vi "No_____Auto_Routine_LeftTrialPieceTRAJ.vi"   [LabVIEW 2023]
uses:
  Shoulder/ShoulderGetSetpointEnum.ctl
  Trajectory/TrajectoryGlobals.vi
  <vilib>/Rock Robotics/WPI/ThirdParty/JAS_Junk/TrajLib/Trajectory_Library.lvlib
types:
  T1 = typedef "ShoulderGetSetpointEnum.ctl" = enum16{"ShoulderRest", "ShoulderShoot", "ShoulderAmp", "ArmFloorPickup", "ArmAmpDeposit", "ArmSpeakerShoot", "ArmStartPosition", "ArmRestPosition", "ArmSourceIntake", "ArmAwayShoot"}
  T2 = typedef "Trajectory_Library.lvlib/TRAJECTORY.ctl" = cluster{"TotalTImeSecs":dbl, "States":T3[]}
  T3 = typedef "Trajectory_Library.lvlib/TRAJ_STATE.ctl" = cluster{"TimeSeconds":dbl, "Velocity":dbl, "Acceleration":dbl, "POSE":T4, "Curvature":dbl}
  T4 = typedef "Trajectory_Library.lvlib/POSE2D.ctl" = cluster{"TRANSLATION":T5, "ROTATION":T6}
  T5 = typedef "Trajectory_Library.lvlib/TRANSLATION2D.ctl" = cluster{"X":dbl, "Y":dbl}
  T6 = typedef "Trajectory_Library.lvlib/ROTATION2D.ctl" = cluster{"VALUE":dbl, "COS":dbl, "SIN":dbl}
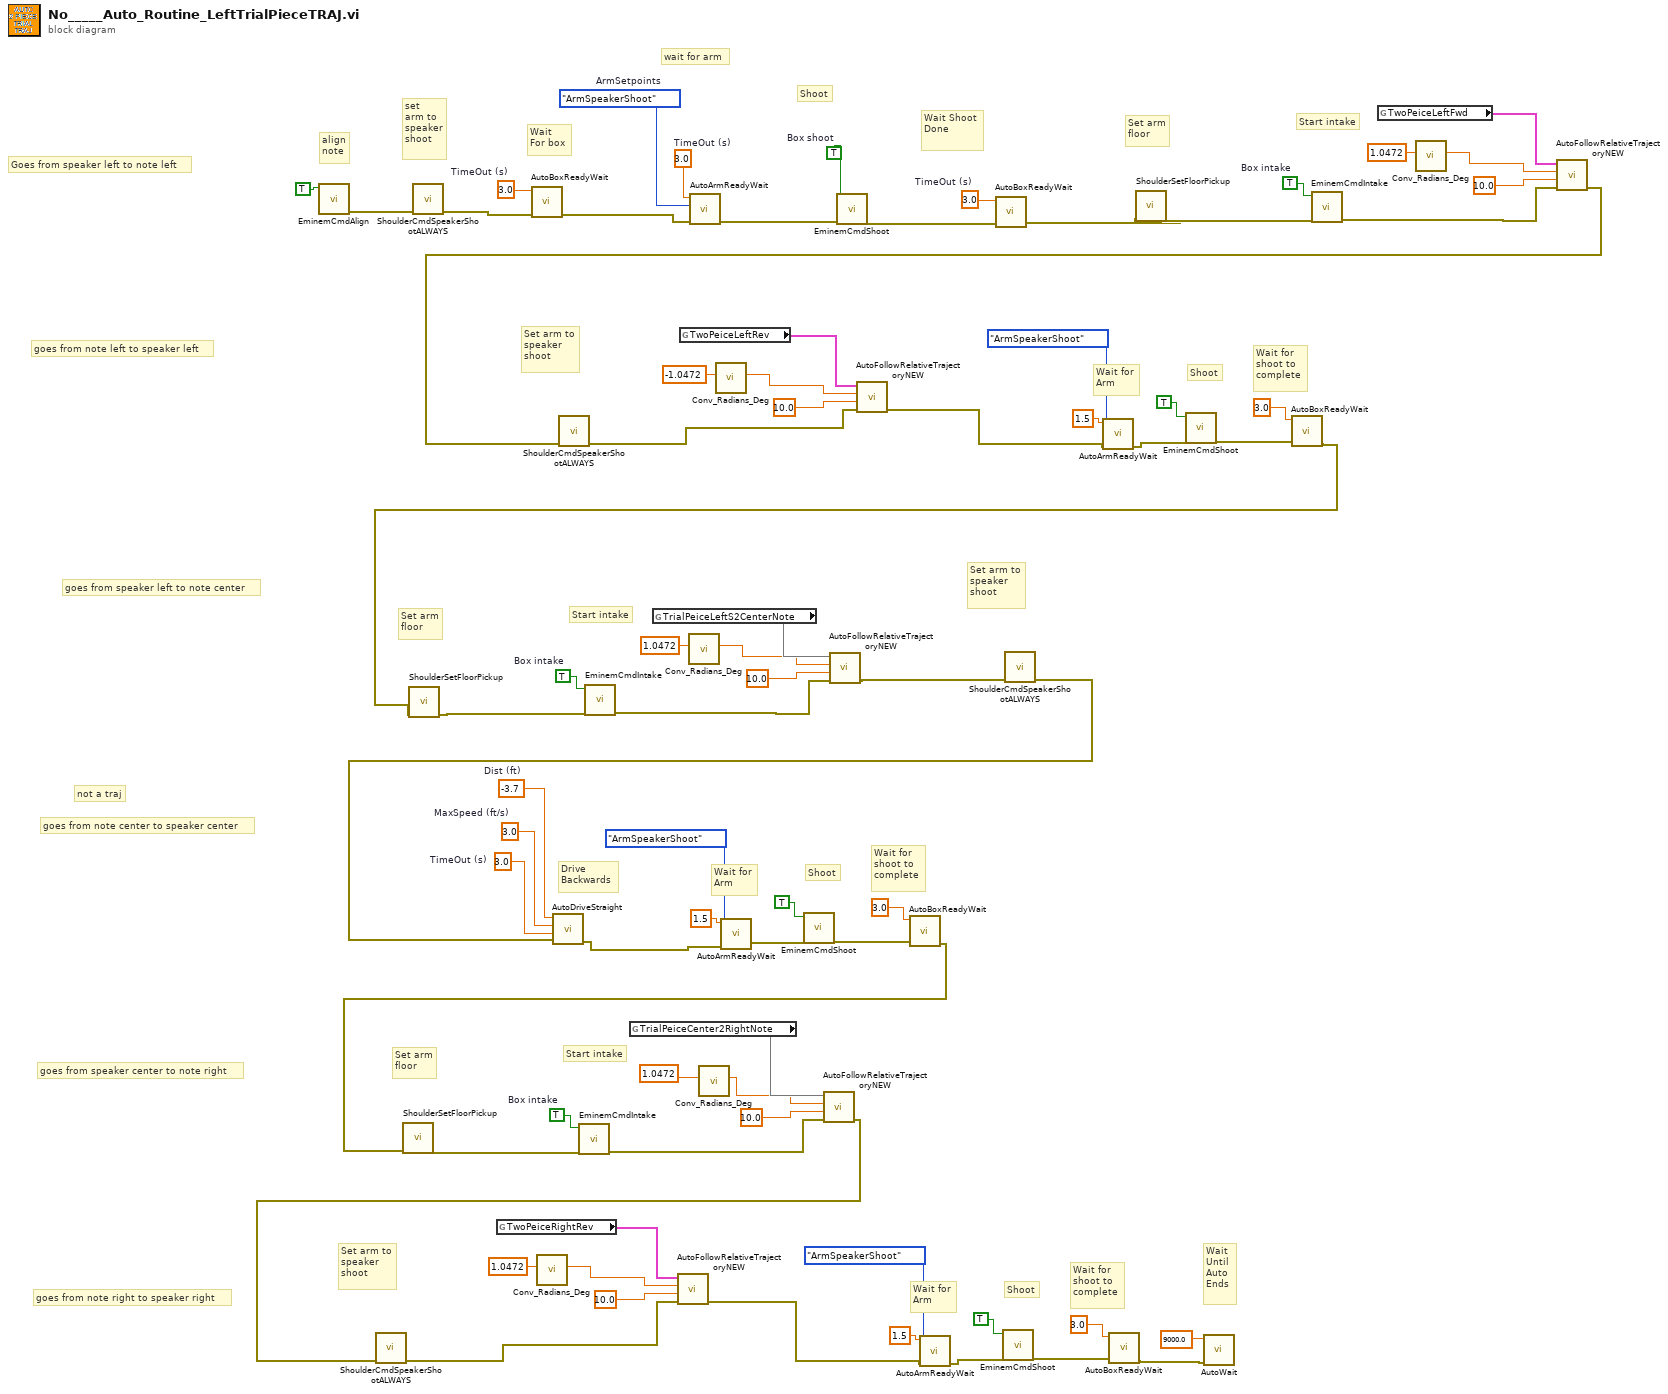
[diagram p0: block diagram]
diagram:
  w23 = TRUE  # Box intake
  w31 = 3.0  # TimeOut (s)
  w30 = 3.0  # MaxSpeed (ft/s)
  w29 = -3.7  # Dist (ft)
  w43 = TRUE  # Box intake
  w65 = 3.0  # TimeOut (s)
  w75 = TRUE  # Box intake
  w74 = TRUE  # Box shoot
  w73 = ShoulderGetSetpointEnum."ArmSpeakerShoot"  # ArmSetpoints
  w72 = 3.0  # TimeOut (s)
  w68 = 3.0  # TimeOut (s)
  # "Wait\nUntil\nAuto \nEnds"
  # "Wait for\nshoot to\ncomplete"
  # "Shoot"
  # "Wait for\nArm"
  # "Set arm to\nspeaker \nshoot"
  # "Start intake"
  # "Set arm\nfloor"
  # "not a traj"
  # "Wait for\nshoot to\ncomplete"
  # "Shoot"
  # "Wait for\nArm"
  # "Drive\nBackwards"
  # "Set arm to\nspeaker \nshoot"
  # "Start intake"
  # "Set arm\nfloor"
  # "goes from note right to speaker right"
  # "goes from speaker center to note right"
  # "goes from note center to speaker center"
  # "goes from speaker left to note center"
  # "goes from note left to speaker left"
  # "Goes from speaker left to note left"
  # "Wait for\nshoot to\ncomplete"
  # "Shoot"
  # "Wait for\nArm"
  # "Set arm to\nspeaker \nshoot"
  # "Start intake"
  # "Set arm\nfloor"
  # "Wait Shoot\nDone"
  # "Shoot"
  # "Wait\nFor box"
  # "set \narm to\nspeaker\nshoot"
  # "align\nnote"
  # "wait for arm"
  n1 = call "EminemCmdAlign.vi"("box align"=TRUE) -> ("error out"=w66:errorcluster)  [unwired: 10 in]
  n2 = call "ShoulderCmdSpeakerShootALWAYS.vi"("error in (no error)"=w66) -> ("error out"=w64:errorcluster)  [unwired: 10 in]
  n3 = global read "TrajectoryGlobals.vi" "TwoPeiceRightRev"() -> (w8:T2)
  n4 = call "AutoBoxReadyWait.vi"("error in (no error)"=w64, "TimeOut (s)"=w65) -> ("error out"=w63:errorcluster)  [unwired: 9 in]
  n5 = call <vilib>:"Conv_Radians_Deg.vi"("Radians"=1.0472) -> ("Degrees"=w6:dbl)  [unwired: 10 in]
  n6 = global read "TrajectoryGlobals.vi" "TrialPeiceCenter2RightNote"() -> (w20)
  n7 = global read "TrajectoryGlobals.vi" "TrialPeiceLeftS2CenterNote"() -> (w41)
  n8 = global read "TrajectoryGlobals.vi" "TwoPeiceLeftRev"() -> (w49:T2)
  n9 = call <vilib>:"Conv_Radians_Deg.vi"("Radians"=1.0472) -> ("Degrees"=w39:dbl)  [unwired: 10 in]
  n10 = call "AutoArmReadyWait.vi"("error in (no error)"=w63, "ArmSetpoints"=w73, "TimeOut (s)"=w72) -> ("error out"=w69:errorcluster)  [unwired: 8 in]
  n11 = call <vilib>:"Conv_Radians_Deg.vi"("Radians"=1.0472) -> ("Degrees"=w18:dbl)  [unwired: 10 in]
  n12 = call <vilib>:"Conv_Radians_Deg.vi"("Radians"=-1.0472) -> ("Degrees"=w47:dbl)  [unwired: 10 in]
  n13 = call "EminemCmdShoot.vi"("error in (no error)"=w69, 11:w74) -> ("error out"=w70:errorcluster)  [unwired: 9 in]
  n14 = call "AutoBoxReadyWait.vi"("error in (no error)"=w70, "TimeOut (s)"=w68) -> ("error out"=w62:errorcluster)  [unwired: 9 in]
  n15 = call "ShoulderSetFloorPickup.vi"("error in (no error)"=w62) -> ("error out"=w71:errorcluster)  [unwired: 10 in]
  n16 = call "EminemCmdIntake.vi"("error in (no error)"=w71, "Box intake"=w75) -> ("error out"=w61:errorcluster)  [unwired: 9 in]
  n17 = global read "TrajectoryGlobals.vi" "TwoPeiceLeftFwd"() -> (w60:T2)
  n18 = call <vilib>:"Conv_Radians_Deg.vi"("Radians"=1.0472) -> ("Degrees"=w58:dbl)  [unwired: 10 in]
  n19 = call "AutoFollowRelativeTrajectoryNEW.vi"("error in (no error)"=w61, "TimeOut (s)"=10.0, "End Orientation"=w58, "Trajectory"=w60) -> ("error out"=w56:errorcluster)  [unwired: 7 in]
  n20 = call "ShoulderCmdSpeakerShootALWAYS.vi"("error in (no error)"=w56) -> ("error out"=w45:errorcluster)  [unwired: 10 in]
  n21 = call "AutoFollowRelativeTrajectoryNEW.vi"("error in (no error)"=w45, "TimeOut (s)"=10.0, "End Orientation"=w47, "Trajectory"=w49) -> ("error out"=w44:errorcluster)  [unwired: 7 in]
  n22 = call "AutoArmReadyWait.vi"("error in (no error)"=w44, "ArmSetpoints"=ShoulderGetSetpointEnum."ArmSpeakerShoot", "TimeOut (s)"=1.5) -> ("error out"=w51:errorcluster)  [unwired: 8 in]
  n23 = call "EminemCmdShoot.vi"("error in (no error)"=w51, 11:TRUE ("Box shoot")) -> ("error out"=w54:errorcluster)  [unwired: 9 in]
  n24 = call "AutoBoxReadyWait.vi"("error in (no error)"=w54, "TimeOut (s)"=3.0) -> ("error out"=w36:errorcluster)  [unwired: 9 in]
  n25 = call "ShoulderSetFloorPickup.vi"("error in (no error)"=w36) -> ("error out"=w37:errorcluster)  [unwired: 10 in]
  n26 = call "EminemCmdIntake.vi"("error in (no error)"=w37, "Box intake"=w43) -> ("error out"=w42:errorcluster)  [unwired: 9 in]
  n27 = call "AutoFollowRelativeTrajectoryNEW.vi"("error in (no error)"=w42, "TimeOut (s)"=10.0, "End Orientation"=w39, "Trajectory"=w41) -> ("error out"=w35:errorcluster)  [unwired: 7 in]
  n28 = call "ShoulderCmdSpeakerShootALWAYS.vi"("error in (no error)"=w35) -> ("error out"=w24:errorcluster)  [unwired: 10 in]
  n29 = call "AutoDriveStraight.vi"("error in (no error)"=w24, "TimeOut (s)"=w31, "MaxSpeed (ft/s)"=w30, "Dist (ft)"=w29) -> ("error out"=w32:errorcluster)  [unwired: 7 in]
  n30 = call "AutoArmReadyWait.vi"("error in (no error)"=w32, "ArmSetpoints"=ShoulderGetSetpointEnum."ArmSpeakerShoot", "TimeOut (s)"=1.5) -> ("error out"=w26:errorcluster)  [unwired: 8 in]
  n31 = call "EminemCmdShoot.vi"("error in (no error)"=w26, 11:TRUE ("Box shoot")) -> ("error out"=w33:errorcluster)  [unwired: 9 in]
  n32 = call "AutoBoxReadyWait.vi"("error in (no error)"=w33, "TimeOut (s)"=3.0) -> ("error out"=w16:errorcluster)  [unwired: 9 in]
  n33 = call "ShoulderSetFloorPickup.vi"("error in (no error)"=w16) -> ("error out"=w22:errorcluster)  [unwired: 10 in]
  n34 = call "EminemCmdIntake.vi"("error in (no error)"=w22, "Box intake"=w23) -> ("error out"=w21:errorcluster)  [unwired: 9 in]
  n35 = call "AutoFollowRelativeTrajectoryNEW.vi"("error in (no error)"=w21, "TimeOut (s)"=10.0, "End Orientation"=w18, "Trajectory"=w20) -> ("error out"=w1:errorcluster)  [unwired: 7 in]
  n36 = call "ShoulderCmdSpeakerShootALWAYS.vi"("error in (no error)"=w1) -> ("error out"=w4:errorcluster)  [unwired: 10 in]
  n37 = call "AutoFollowRelativeTrajectoryNEW.vi"("error in (no error)"=w4, "TimeOut (s)"=10.0, "End Orientation"=w6, "Trajectory"=w8) -> ("error out"=w3:errorcluster)  [unwired: 7 in]
  n38 = call "AutoArmReadyWait.vi"("error in (no error)"=w3, "ArmSetpoints"=ShoulderGetSetpointEnum."ArmSpeakerShoot", "TimeOut (s)"=1.5) -> ("error out"=w11:errorcluster)  [unwired: 8 in]
  n39 = call "EminemCmdShoot.vi"("error in (no error)"=w11, 11:TRUE ("Box shoot")) -> ("error out"=w14:errorcluster)  [unwired: 9 in]
  n40 = call "AutoBoxReadyWait.vi"("error in (no error)"=w14, "TimeOut (s)"=3.0) -> ("error out"=w2:errorcluster)  [unwired: 9 in]
  n41 = call "AutoWait.vi"("error in (no error)"=w2, "TimeOut (s)"=9000.0) -> ()  [unwired: 9 in, 1 out]
